vi "Modules - Instrument _ Calibration.vi"(8 "error in":errorcluster) -> (0 "error out":errorcluster)   [LabVIEW 2019]
uses:
  Controls/InstrumentCalibraton - State.ctl
  Controls/FGV States.ctl
  <vilib>/Utility/miscctls.llb/LVRowAndColumnTypeDef.ctl
  Controls/eFGV States.ctl
panel:
  in  "Reset Zero":bool
  in  "Zeroing":bool
  out "subarray":string[](array[string])
  in  "OK":bool
  in  "Remove":bool
  in  "Add":bool
  out "Table":string[][](table)
  # "*Select Row to ZEROING"
  # "*Double-Click to Edit"
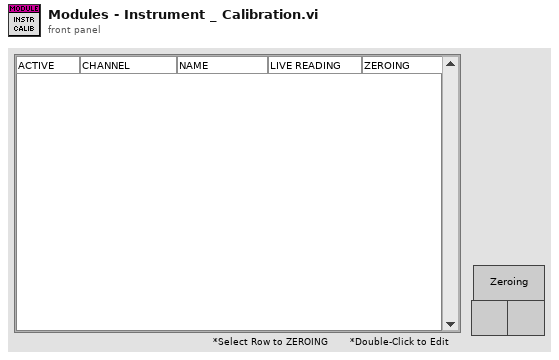
[diagram p1: front panel]
types:
  T1 = typedef "InstrumentCalibraton - State.ctl" = enum16{"Init", "Idle", "Read sensor", "Read DB", "Add", "Edit", "Zero", "Reset Zero", "Remove", "Close", "Exit"}
  T2 = typedef "FGV States.ctl" = enum16{"Read", "Write"}
  T3 = enum32{"Invalid", "Standard", "Closed", "Hidden", "Minimized", "Maximized"}
  T4 = typedef "eFGV States.ctl" = enum16{"Init", "Read", "Write", "Exit"}
  T5 = typedef "LVRowAndColumnTypeDef.ctl" = cluster{"Row":i32, "Column":i32}
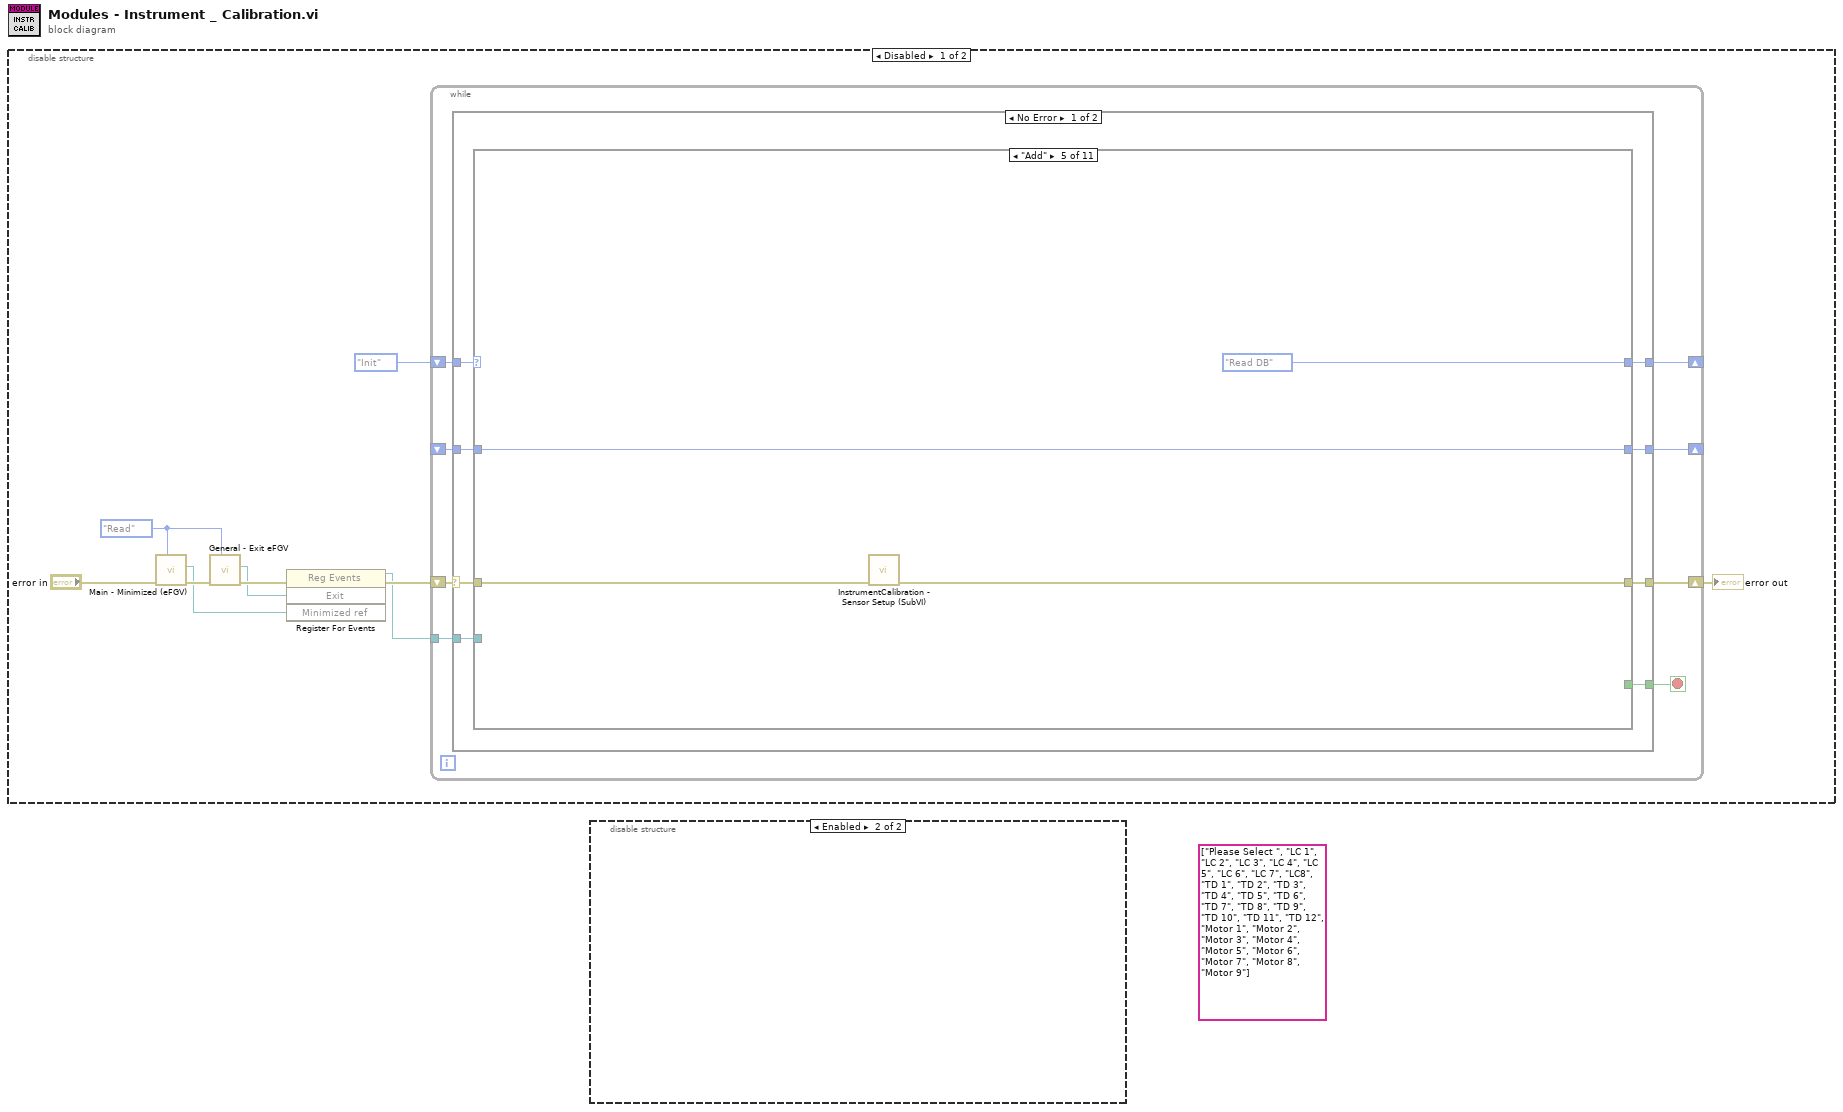
[diagram p0: block diagram]
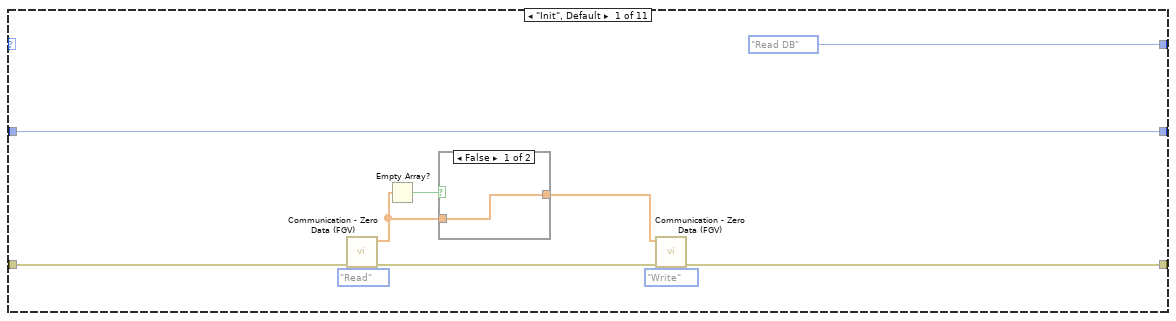
[diagram p2: hidden frame]
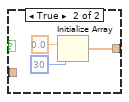
[diagram p3: hidden frame]
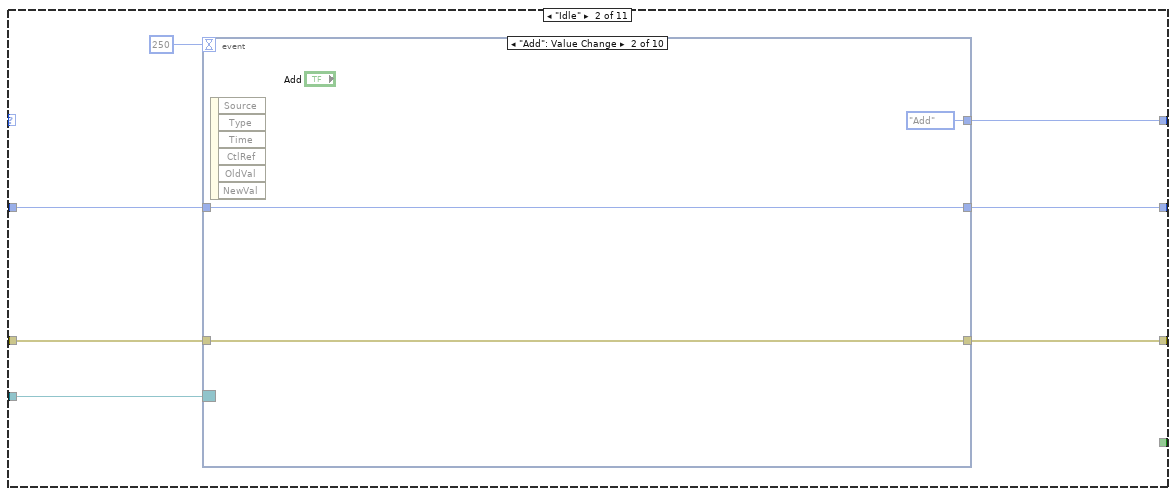
[diagram p4: hidden frame]
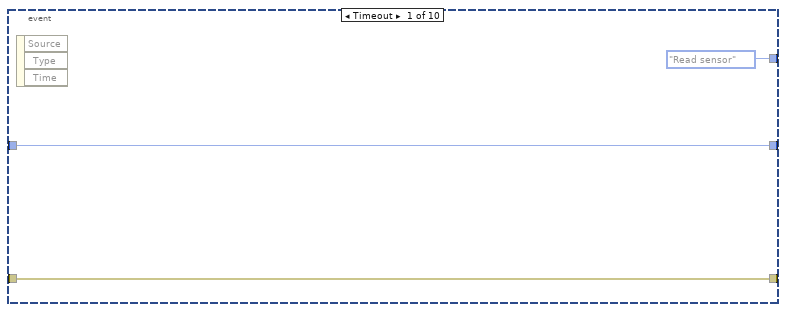
[diagram p5: hidden frame]
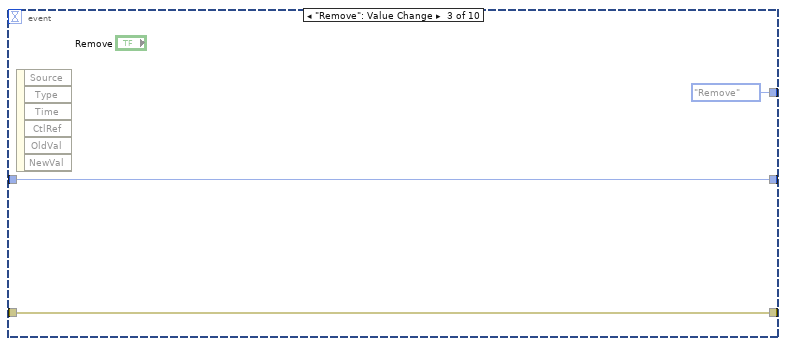
[diagram p6: hidden frame]
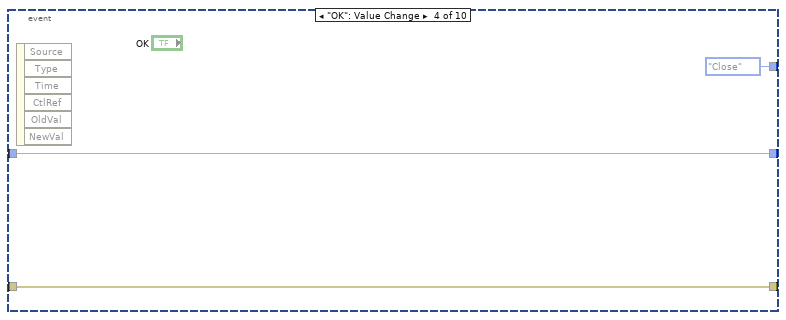
[diagram p7: hidden frame]
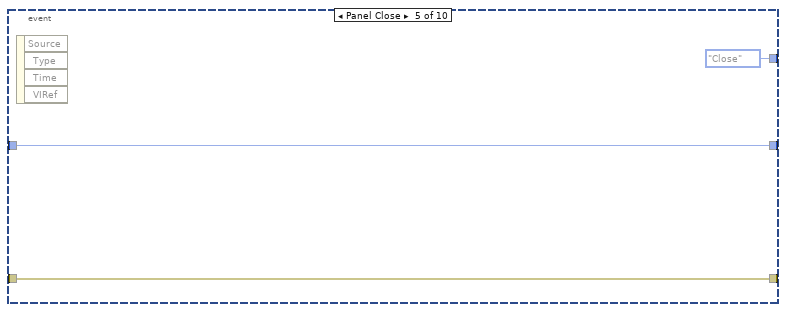
[diagram p8: hidden frame]
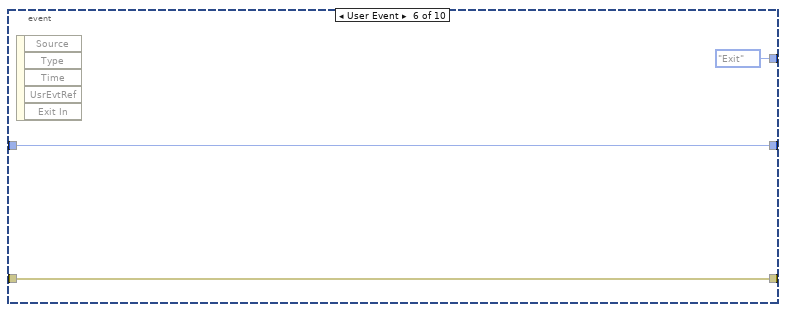
[diagram p9: hidden frame]
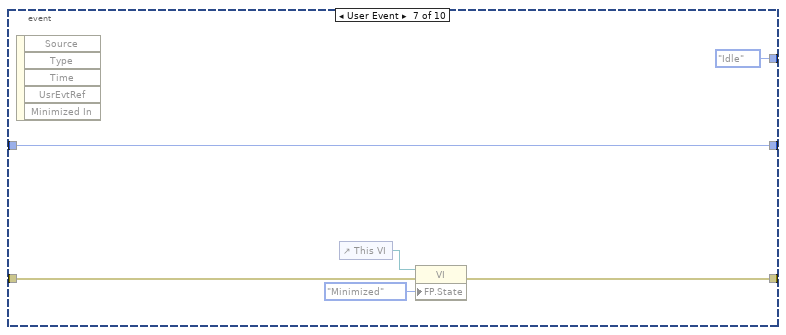
[diagram p10: hidden frame]
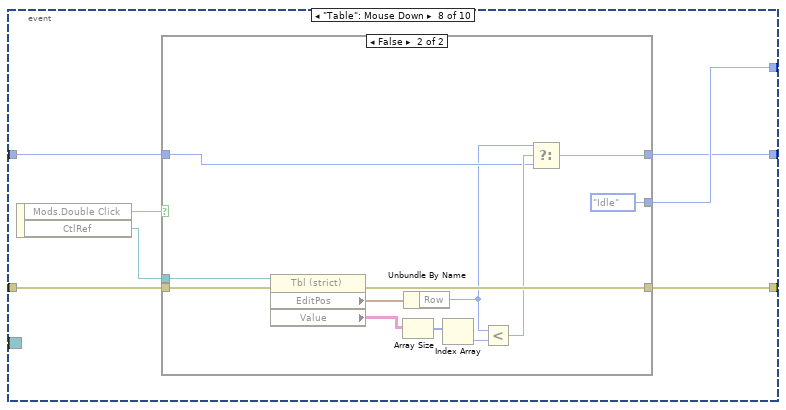
[diagram p11: hidden frame]
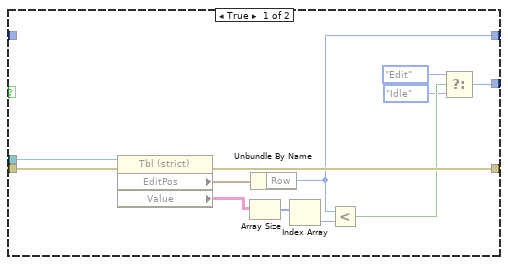
[diagram p12: hidden frame]
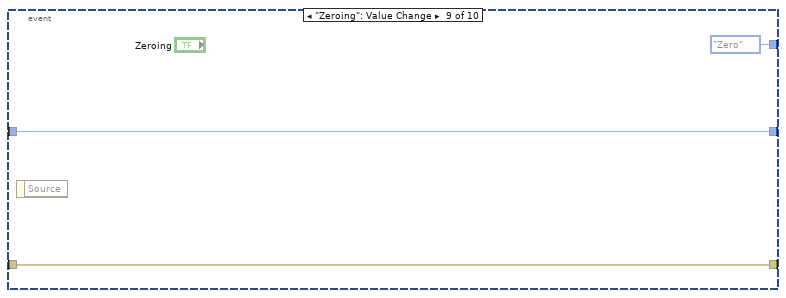
[diagram p13: hidden frame]
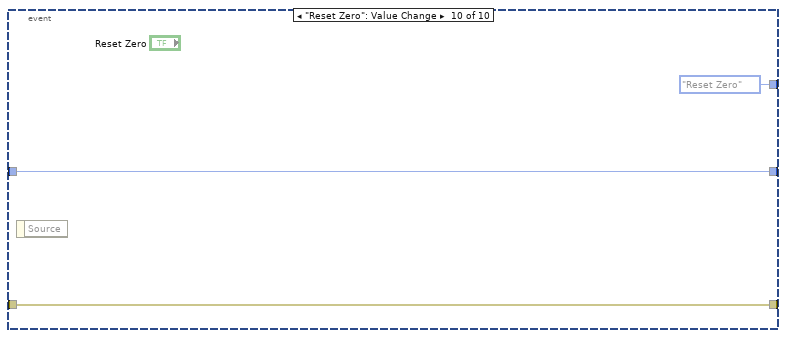
[diagram p14: hidden frame]
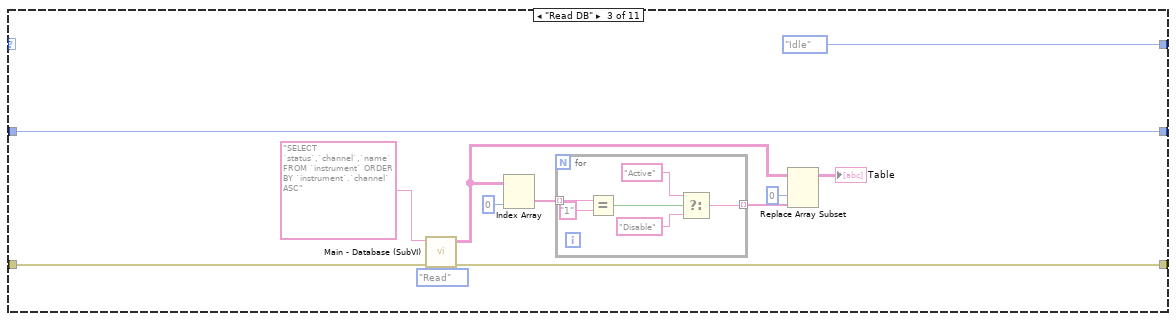
[diagram p15: hidden frame]
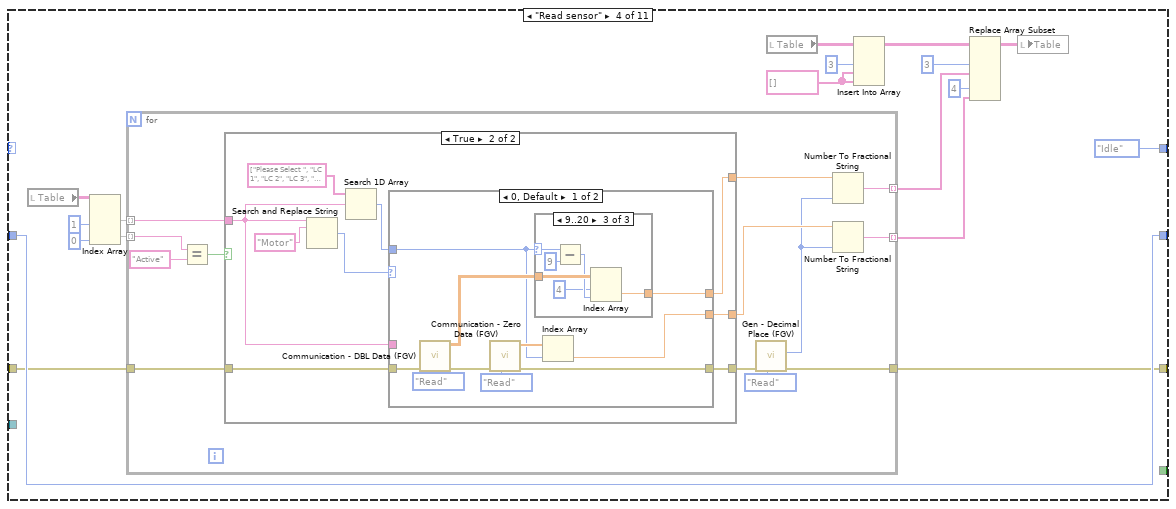
[diagram p16: hidden frame]
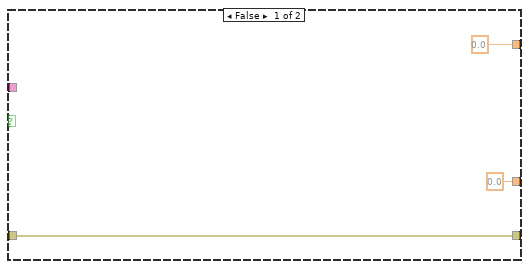
[diagram p17: hidden frame]
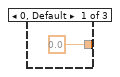
[diagram p18: hidden frame]
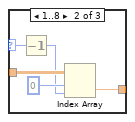
[diagram p19: hidden frame]
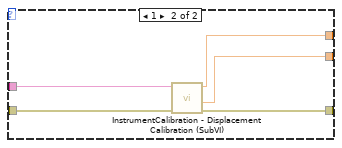
[diagram p20: hidden frame]
diagram:
  (unwired) string[] ["Please Select ", "LC 1", "LC 2", "LC 3", "LC 4", "LC 5", "LC 6", "LC 7", "LC8", "TD 1", "TD 2", "TD 3", "TD 4", "TD 5", "TD 6", "TD 7", "TD 8", "TD 9", "TD 10", "TD 11", "TD 12", "Motor 1", "Motor 2", "Motor 3", "Motor 4", "Motor 5", "Motor 6", "Motor 7", "Motor 8", "Motor 9"] ("string")
  n1 = disable-structure shown="Disabled" {
    frame Disabled {
      w2 = eFGV_States."Read" ("eFGV States")
      n2 = call "Main - Minimized (eFGV).vi"("Action"=w2, "error in"="error in") -> ("error out"=w3:errorcluster, "Minimized ref"=w1:refnum<user-event>)  [unwired: 7 in, 1 out]
      n3 = call "General - Exit eFGV.vi"("eFGV States"=w2, "error in (no error)"=w3) -> ("error out"=w8:errorcluster, "Exit"=w6:refnum<user-event>)  [unwired: 7 in, 1 out]
      n4 = register-events(error in=w8, w6, w1) -> (reference out=w5:refnum<event-registration>, error out=w7:errorcluster)  [unwired: 1 in]
      n5 = while {
        shift-right: [w17] -> w10
        shift-left: w7 -> [w18]
        shift-right: [w15] -> _
        shift-left: InstrumentCalibraton_-_State."Init" -> [w16]
        shift-right: [w13] -> _
        shift-left: _ -> [w12]
        tunnel: w5 -> [w11]
        stop <- w14 stop-if-true
        n6 = case shown="No Error" w18 {
          selector: w18 -> [w25 w282]
          tunnel: [w26 w281] -> w17
          tunnel: w16 -> [w24 _]
          tunnel: [w23 InstrumentCalibraton_-_State."Idle"] -> w15
          tunnel: [w22 _] -> w14
          tunnel: [w21 w278] -> w13
          tunnel: w12 -> [w20 w278]
          tunnel: w11 -> [w19 _]
          frame No Error {
            n7 = case shown="\"Add\"" w24 {
              tunnel: [w27 w47 w118 w134 w199 w206 w223 w244 w263 w267 w274] -> w26
              tunnel: w25 -> [w31 w46 w117 w140 w198 w204 w212 w250 w262 w266 w273]
              tunnel: [InstrumentCalibraton_-_State."Read DB" w45 InstrumentCalibraton_-_State."Idle" InstrumentCalibraton_-_State."Idle" InstrumentCalibraton_-_State."Read DB" InstrumentCalibraton_-_State."Read DB" InstrumentCalibraton_-_State."Idle" InstrumentCalibraton_-_State."Idle" InstrumentCalibraton_-_State."Read DB" InstrumentCalibraton_-_State."Idle" InstrumentCalibraton_-_State."Exit"] -> w23
              tunnel: [_ _ _ _ _ _ _ _ _ _ TRUE] -> w22
              tunnel: [w35 w44 w115 w143 w197 w205 0 ("Row") 0 ("Row") w260 w265 w275] -> w21
              tunnel: w20 -> [w35 w43 w115 w143 w197 w205 w222 w241 w260 w265 w275]
              tunnel: w19 -> [_ w41 _ _ _ _ _ _ _ _ _]
              frame "Init", Default {
                n8 = call "Communication - Zero Data (FGV).vi"("Action"=FGV_States."Read", "error in (no error)"=w31) -> ("error out"=w29:errorcluster, "Zero Out"=w32:dbl[])  [unwired: 8 in]
                n9 = Empty Array?(array=w32) -> (empty?=w33:bool)
                n10 = case shown="False" w33 {
                  tunnel: [w37 w38] -> w28
                  tunnel: w32 -> [w37 _]
                  frame False {
                  }
                  frame True {
                    n11 = Initialize Array(0.0 ("element"), 30 ("dimension size")) -> (w38:dbl[])
                  }
                }
                n12 = call "Communication - Zero Data (FGV).vi"("Action"=FGV_States."Write", "error in (no error)"=w29, "Zero"=w28) -> ("error out"=w27:errorcluster)  [unwired: 7 in, 1 out]
              }
              frame "Idle" {
                n13 = event shown="[1] \"Add\": Value Change" {
                  selector: w41 -> [_ _ _ _ _ _ _ _ _ _]
                  dyn-events: _ -> [_ _ _ _ _ _ _ _ _ _]
                  timeout: 250 -> [_ _ _ _ _ _ _ _ _ _]
                  tunnel: [w50 w53 w56 w59 w62 w65 w67 w78 w103 w106] -> w47
                  tunnel: w46 -> [w50 w53 w56 w59 w62 w65 w68 w77 w103 w106]
                  tunnel: [InstrumentCalibraton_-_State."Read sensor" InstrumentCalibraton_-_State."Add" InstrumentCalibraton_-_State."Remove" InstrumentCalibraton_-_State."Close" InstrumentCalibraton_-_State."Close" InstrumentCalibraton_-_State."Exit" InstrumentCalibraton_-_State."Idle" ("f") w74 InstrumentCalibraton_-_State."Zero" ("f") InstrumentCalibraton_-_State."Reset Zero" ("f")] -> w45
                  tunnel: [w48 w51 w54 w57 w60 w63 w71 w73 w105 w108] -> w44
                  tunnel: w43 -> [w48 w51 w54 w57 w60 w63 w71 w72 w105 w108]
                  event Timeout {
                    n14 = event-data() -> ()  [unwired: 1 in, 3 out]
                  }
                  event "Add": Value Change {
                    n15 = event-data() -> ()  [unwired: 1 in, 6 out]
                  }
                  event "Remove": Value Change {
                    n16 = event-data() -> ()  [unwired: 1 in, 6 out]
                  }
                  event "OK": Value Change {
                    n17 = event-data() -> ()  [unwired: 1 in, 6 out]
                  }
                  event Panel Close {
                    n18 = event-data() -> ()  [unwired: 1 in, 4 out]
                  }
                  event User Event {
                    n19 = event-data() -> ()  [unwired: 1 in, 5 out]
                  }
                  event User Event {
                    n20 = event-data() -> ()  [unwired: 1 in, 5 out]
                    n21 = control-ref of="This VI"() -> (w70:refnum<vi>)
                    n22 = property class="VI"(reference=w70, error in=w68, "FP.State"=T3."Minimized" ("Front Panel Window:State")) -> (error out=w67:errorcluster)  [unwired: 1 out]
                  }
                  event "Table": Mouse Down {
                    n23 = event-data() -> ("Mods.Double Click"=w75:bool, "CtlRef"=w76:refnum<vi>)  [unwired: 1 in]
                    n24 = case shown="False" w75 {
                      tunnel: [w90 w102] -> w78
                      tunnel: w77 -> [w89 w101]
                      tunnel: w76 -> [w88 w100]
                      tunnel: [w82 InstrumentCalibraton_-_State."Idle" ("f")] -> w74
                      tunnel: [w80 w91] -> w73
                      tunnel: w72 -> [_ w94]
                      frame True {
                        n25 = property class="Tbl (strict)"(reference=w88, error in=w89) -> (error out=w90:errorcluster, "EditPos"=w87:T5, "Value"=w79:string[][])  [unwired: 1 out]
                        n26 = Array Size(array=w79) -> (size(s)=w86:i32[])
                        n27 = Unbundle By Name(w87) -> ("Row"=w80:i32)
                        n28 = Index Array(array=w86) -> (element=w85:i32)  [unwired: 1 in]
                        n29 = Less?(x=w80, y=w85) -> (x < y?=w84:bool)
                        n30 = Select(t=InstrumentCalibraton_-_State."Edit", s=w84, f=InstrumentCalibraton_-_State."Idle") -> (s? t:f=w82:T1)
                      }
                      frame False {
                        n31 = property class="Tbl (strict)"(reference=w100, error in=w101) -> (error out=w102:errorcluster, "EditPos"=w99:T5, "Value"=w95:string[][])  [unwired: 1 out]
                        n32 = Array Size(array=w95) -> (size(s)=w98:i32[])
                        n33 = Unbundle By Name(w99) -> ("Row"=w92:i32)
                        n34 = Index Array(array=w98) -> (element=w97:i32)  [unwired: 1 in]
                        n35 = Less?(x=w92, y=w97) -> (x < y?=w96:bool)
                        n36 = Select(t=w92, s=w96, f=w94) -> (s? t:f=w91:i32)
                      }
                    }
                  }
                  event "Zeroing": Value Change {
                    n37 = event-data() -> ()  [unwired: 1 in, 1 out]
                  }
                  event "Reset Zero": Value Change {
                    n38 = event-data() -> ()  [unwired: 1 in, 1 out]
                  }
                }
              }
              frame "Read DB" {
                n39 = call "Main - Database (SubVI).vi"("Enum"=FGV_States."Read", "error in (no error)"=w117, "SQL query"="SELECT `status`,`channel`,`name` FROM `instrument` ORDER BY `instrument`.`channel` ASC") -> ("error out"=w118:errorcluster, "data"=w112:string[][])  [unwired: 7 in]
                n40 = Index Array(array=w112, index (col)=0 ("disabled index (col)")) -> (element=w113:string[])  [unwired: 1 in]
                n41 = for {
                  tunnel: w113 -> [w126] mode=indexing
                  tunnel: [w121] -> w110 mode=indexing
                  n42 = Equal?(x=w126, y="1") -> (x = y?=w124:bool)
                  n43 = Select(t="Active" ("y"), s=w124, f="Disable" ("y")) -> (s? t:f=w121:string)
                }
                n44 = Replace Array Subset(array=w112, new element=w110, index (col)=0 ("disabled index (col)")) -> (→"Table":string[][])  [unwired: 1 in]
              }
              frame "Read sensor" {
                w127 = string[] [] ("new element/subarray")
                n45 = local read "Table"() -> (w142:string[][])
                n46 = Index Array(array=w142, index (col) #1=1 ("disabled index (col)"), index (col) #2=0 ("index (col)")) -> (element #1=w139:string[], element #2=w132:string[])  [unwired: 2 in]
                n47 = for {
                  tunnel: w139 -> [w149] mode=indexing
                  tunnel: w140 -> [w157]
                  tunnel: [w150] -> w134
                  tunnel: w132 -> [w156] mode=indexing
                  tunnel: [w148] -> w131 mode=indexing
                  tunnel: [w146] -> w130 mode=indexing
                  n48 = Equal?(x=w156, y="Active") -> (x = y?=w154:bool)
                  n49 = case shown="True" w154 {
                    tunnel: w149 -> [_ w163]
                    tunnel: w157 -> [w160 w167]
                    tunnel: [w160 w166] -> w151
                    tunnel: [0.0 ("shared variable refnum in") w164] -> w152
                    tunnel: [0.0 ("shared variable refnum in") w161] -> w147
                    frame False {
                    }
                    frame True {
                      n50 = Search and Replace String(input string=w163, search string="Motor") -> (number of replacements=w168:i32)  [unwired: 6 in, 3 out]
                      n51 = Search 1D Array(1D array=string[] ["Please Select ", "LC 1", "LC 2", "LC 3", "LC 4", "LC 5", "LC 6", "LC 7", "LC 8", "TD 1", "TD 2", "TD 3", "TD 4", "TD 5", "TD 6", "TD 7", "TD 8", "TD 9", "TD 10", "TD 11", "TD 12", "Motor 1", "Motor 2", "Motor 3", "Motor 4", "Motor 5", "Motor 6", "Motor 7", "Motor 8", "Motor 9"] ("string"), element=w163) -> (index of element=w165:i32)  [unwired: 1 in]
                      n52 = case shown="0, Default" w168 {
                        tunnel: w167 -> [w177 w196]
                        tunnel: [w174 w195] -> w166
                        tunnel: w165 -> [w172 _]
                        tunnel: [w170 w193] -> w164
                        tunnel: w163 -> [_ w194]
                        tunnel: [w171 w192] -> w161
                        frame 0, Default {
                          n53 = call "Communication - DBL Data (FGV).vi"("Action"=FGV_States."Read", "error in (no error)"=w177) -> ("error out"=w175:errorcluster, "DBL SV Out"=w179:dbl[][])  [unwired: 8 in]
                          n54 = call "Communication - Zero Data (FGV).vi"("Action"=FGV_States."Read", "error in (no error)"=w175) -> ("error out"=w174:errorcluster, "Zero Out"=w173:dbl[])  [unwired: 8 in]
                          n55 = case shown="9..20" w172 {
                            selector: w172 -> [_ w184 w189]
                            tunnel: w179 -> [_ w185 w191]
                            tunnel: [0.0 ("shared variable refnum in") w183 w190] -> w170
                            frame 0, Default {
                            }
                            frame 1..8 {
                              n56 = Decrement(x=w184) -> (x-1=w181:i32)
                              n57 = Index Array(array=w185, index (row)=0 ("disabled index (col)"), index (col)=w181) -> (element=w183:dbl)
                            }
                            frame 9..20 {
                              n58 = Subtract(x=w189, y=9 ("disabled index (col)")) -> (x-y=w187:i32)
                              n59 = Index Array(array=w191, index (row)=4 ("disabled index (col)"), index (col)=w187) -> (element=w190:dbl)
                            }
                          }
                          n60 = Index Array(array=w173, index=w172) -> (element=w171:dbl)
                        }
                        frame 1 {
                          n61 = call "InstrumentCalibration - Displacement Calibration (SubVI).vi"("error in (no error)"=w196, "Motor No"=w194) -> ("error out"=w195:errorcluster, "Zero"=w192:dbl, "Displacement"=w193:dbl)  [unwired: 6 in, 1 out]
                        }
                      }
                    }
                  }
                  n62 = call "Gen - Decimal Place (FGV).vi"("Action"=FGV_States."Read", "error In"=w151) -> ("error out"=w150:errorcluster, "Ch2 out"=w145:u8)  [unwired: 7 in, 1 out]
                  n63 = Number To Fractional String(number=w152, precision (6)=w145) -> (F-format string=w148:string)  [unwired: 2 in]
                  n64 = Number To Fractional String(number=w147, precision (6)=w145) -> (F-format string=w146:string)  [unwired: 2 in]
                }
                n65 = local read "Table"() -> (w136:string[][])
                n66 = Insert Into Array(array=w136, index (col)=3 ("disabled index (col)"), new element #1=w127, new element #2=w127) -> (w135:string[][])  [unwired: 1 in]
                n67 = Replace Array Subset(array=w135, new element #1=w131, index (col) #1=3 ("disabled index (col)"), new element #2=w130, index (col) #2=4 ("index (col)")) -> (w137:string[][])  [unwired: 2 in]
                n68 = local write "Table"(w137) -> ()
              }
              frame "Add" {
                n69 = call "InstrumentCalibration - Sensor Setup (SubVI).vi"("error in"=w198) -> ("error out"=w199:errorcluster)  [unwired: 10 in]
              }
              frame "Edit" {
                n70 = local read "Table"() -> (w202:string[][])
                n71 = Index Array(array=w202, index (row)=w205) -> (element=w203:string[])  [unwired: 1 in]
                n72 = Index Array(array=w202, index (col)=0 ("disabled index (col)")) -> ()  [unwired: 1 in, 1 out]
                n73 = call "InstrumentCalibration - Sensor Setup (SubVI).vi"("error in"=w204, "Edit"=w203) -> ("error out"=w206:errorcluster)  [unwired: 9 in]
              }
              frame "Zero" {
                n74 = local read "Table"() -> (w230:string[][])
                n75 = Index Array(array=w230, index (row) #1=w222, index (col) #1=1 ("disabled index (col)"), index (row) #2=w222, index (col) #2=3 ("disabled index (col)")) -> (element #1=w208:string, element #2=w219:string)
                n76 = Fract/Exp String To Number(string=w219) -> (number=w210:dbl)  [unwired: 3 in, 1 out]
                n77 = Search 1D Array(1D array=string[] ["Please Select ", "LC 1", "LC 2", "LC 3", "LC 4", "LC 5", "LC 6", "LC 7", "LC 8", "TD 1", "TD 2", "TD 3", "TD 4", "TD 5", "TD 6", "TD 7", "TD 8", "TD 9", "TD 10", "TD 11", "TD 12", "Motor 1", "Motor 2", "Motor 3", "Motor 4", "Motor 5", "Motor 6", "Motor 7", "Motor 8", "Motor 9"] ("string"), element=w208) -> (index of element=w209:i32)  [unwired: 1 in]
                n78 = Search and Replace String(input string=w208, search string="Motor") -> (number of replacements=w214:i32)  [unwired: 6 in, 3 out]
                n79 = case shown="0, Default" w214 {
                  tunnel: [w233 w234] -> w213
                  tunnel: w212 -> [w233 w237]
                  tunnel: [w232 w235] -> w211
                  tunnel: w210 -> [w232 _]
                  tunnel: w209 -> [_ _]
                  tunnel: w208 -> [_ w236]
                  frame 0, Default {
                  }
                  frame 1 {
                    n80 = call "InstrumentCalibration - Displacement Calibration (SubVI).vi"("error in (no error)"=w237, "Motor No"=w236) -> ("error out"=w234:errorcluster, "Displacement"=w235:dbl)  [unwired: 6 in, 2 out]
                  }
                }
                n81 = call "Communication - Zero Data (FGV).vi"("Action"=FGV_States."Read", "error in (no error)"=w213) -> ("error out"=w224:errorcluster, "Zero Out"=w226:dbl[])  [unwired: 8 in]
                n82 = Index Array(array=w226, index=w209) -> (element=w217:dbl)
                n83 = Add(x=w217, y=w211) -> (x+y=w216:dbl)
                n84 = Replace Array Subset(array=w226, new element=w216, index=w209) -> (w218:dbl[])
                n85 = call "Communication - Zero Data (FGV).vi"("Action"=FGV_States."Write", "error in (no error)"=w224, "Zero"=w218) -> ("error out"=w223:errorcluster)  [unwired: 7 in, 1 out]
              }
              frame "Reset Zero" {
                n86 = local read "Table"() -> (w254:string[][])
                n87 = Index Array(array=w254, index (row)=w241, index (col)=1 ("disabled index (col)")) -> (element=w251:string)
                n88 = call "Communication - Zero Data (FGV).vi"("Action"=FGV_States."Read", "error in (no error)"=w250) -> ("error out"=w245:errorcluster, "Zero Out"=w247:dbl[])  [unwired: 8 in]
                n89 = Search 1D Array(1D array=string[] ["Please Select ", "LC 1", "LC 2", "LC 3", "LC 4", "LC 5", "LC 6", "LC 7", "LC 8", "TD 1", "TD 2", "TD 3", "TD 4", "TD 5", "TD 6", "TD 7", "TD 8", "TD 9", "TD 10", "TD 11", "TD 12", "Motor 1", "Motor 2", "Motor 3", "Motor 4", "Motor 5", "Motor 6", "Motor 7", "Motor 8", "Motor 9"] ("string"), element=w251) -> (index of element=w242:i32)  [unwired: 1 in]
                n90 = Empty Array?(array=w247) -> (empty?=w248:bool)
                n91 = case shown="True" w248 {
                  tunnel: [w256 w257] -> w243
                  tunnel: w247 -> [w256 _]
                  frame False {
                  }
                  frame True {
                    n92 = Initialize Array(0.0 ("element"), 30 ("dimension size")) -> (w257:dbl[])
                  }
                }
                n93 = Replace Array Subset(array=w243, new element=0.0 ("new element/subarray"), index=w242) -> (w239:dbl[])
                n94 = call "Communication - Zero Data (FGV).vi"("Action"=FGV_States."Write", "error in (no error)"=w245, "Zero"=w239) -> ("error out"=w244:errorcluster)  [unwired: 7 in, 1 out]
              }
              frame "Remove" {
                n95 = local read "Table"() -> (w261:string[][])
                n96 = call "InstrumentCalibration - Remove Channel (SubVI).vi"("error in"=w262, "Table"=w261) -> ("error out"=w263:errorcluster)  [unwired: 7 in, 2 out]
              }
              frame "Close" {
                n97 = control-ref of="This VI"() -> (w270:refnum<vi>)
                n98 = invoke class="VI" method="FP.Close"(reference=w270, error in=w266) -> (reference out=w268:refnum<vi>, error out=w269:errorcluster)  [unwired: 1 in, 1 out]
                n99 = Close Reference(reference=w268, error in (no error)=w269) -> (error out=w267:errorcluster)
              }
              frame "Exit" {
                n100 = control-ref of="This VI"() -> (w272:refnum<vi>)
                n101 = invoke class="VI" method="FP.Close"(reference=w272, error in=w273) -> (error out=w274:errorcluster)  [unwired: 1 in, 2 out]
              }
            }
          }
          frame Error {
            n102 = call <vilib>:"Clear Errors.vi"("error in (no error)"=w282) -> ("error out"=w281:errorcluster)  [unwired: 5 in, 1 out]
            n103 = Wait (ms)(milliseconds to wait=u32 100) -> ()  [unwired: 1 out]
          }
        }
      }
      "error out" <- w10
    }
    frame Enabled {
    }
  }
  n104 = disable-structure shown="Enabled" {
    frame Disabled {
      n105 = for {
        N: 100 -> [_]
        tunnel: T5 {"Row"=0, "Column"=-2} ("Active Cell:Active Cell") -> [w292]
        i -> [w291]
        n106 = Bundle By Name(cluster=w292, "Row"=w291) -> (w293:T5)
        n107 = Quotient & Remainder(x=w291, y=2) -> (x-y*floor(x/y)=w289:i32)  [unwired: 1 out]
        n108 = Equal To 0?(x=w289) -> (x = 0?=w288:bool)
        n109 = Select(t=u32 16777238, s=w288, f=u32 16777225) -> (s? t:f=w286:u32)
        n110 = property on="Table" class="Tbl (strict)"("Active Cell"=w293, "Justify"=enum16{"Left", "Center", "Right"}."Center" ("Active Cell:Cell Justification"), "Cell BG Color"=w286) -> ()  [unwired: 2 in, 2 out]
      }
    }
    frame Enabled {
    }
  }
